vi "ConfigureQDC.vi"(5 "VME module Base Address":u32, 6 "IRQ Lvl":u16, 7 "handle":i32, 8 "error in (no error)":errorcluster, 9 "# of events before transfer (max 32)":u16, 10 "CBLT Addr":u16, 11 "Geo Addr":u16) -> (0 "error out":errorcluster, 3 "handle out":i32)   [LabVIEW 2014]
uses:
  Program Files (x86)/CAEN/Comm/labview/CAENComm.lvlib
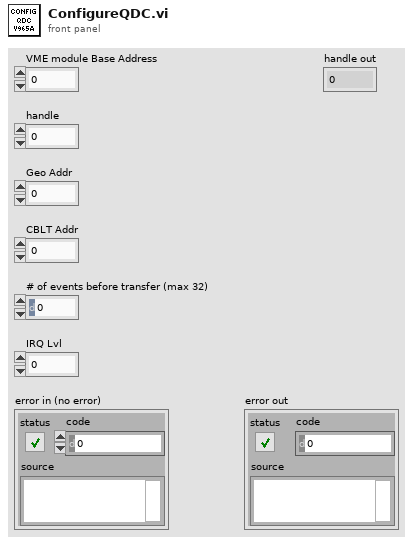
[diagram p1: front panel]
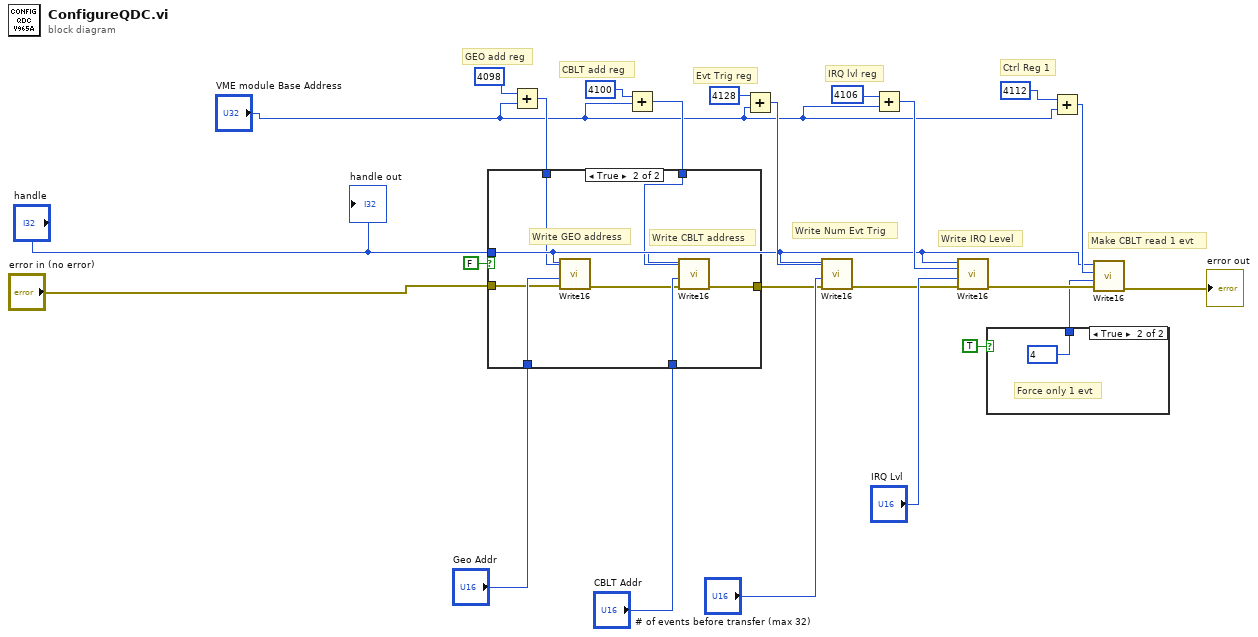
[diagram p0: block diagram]
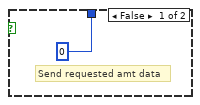
[diagram p2: hidden frame]
diagram:
  # "Ctrl Reg 1"
  # "Make CBLT read 1 evt"
  # "Evt Trig reg"
  # "Write Num Evt Trig"
  # "IRQ lvl reg"
  # "Write IRQ Level"
  # "CBLT add reg"
  # "GEO add reg"
  n1 = Add(x=u32 4098, y="VME module Base Address") -> (x+y=w11:u32)
  n2 = Add(x=u32 4100, y="VME module Base Address") -> (x+y=w15:u32)
  n3 = case shown="True" FALSE {
    tunnel: [w25 w33] -> w17
    tunnel: "CBLT Addr" -> [_ w32]
    tunnel: w15 -> [_ w31]
    tunnel: "Geo Addr" -> [_ w29]
    tunnel: w11 -> [_ w28]
    tunnel: "error in (no error)" -> [w25 w27]
    tunnel: "handle" -> [_ w26]
    frame False {
    }
    frame True {
      # "Write CBLT address"
      # "Write GEO address"
      n4 = call "Write16.vi"("error in (no error)"=w27, "Data"=w29, "Address"=w28, "handle"=w26) -> ("error out"=w30:errorcluster)  [unwired: 7 in]
      n5 = call "Write16.vi"("error in (no error)"=w30, "Data"=w32, "Address"=w31, "handle"=w26) -> ("error out"=w33:errorcluster)  [unwired: 7 in]
    }
  }
  n6 = Add(x=u32 4128, y="VME module Base Address") -> (x+y=w19:u32)
  n7 = call "Write16.vi"("error in (no error)"=w17, "Data"="# of events before transfer (max 32)", "Address"=w19, "handle"="handle") -> ("error out"=w20:errorcluster)  [unwired: 7 in]
  n8 = Add(x=u32 4106, y="VME module Base Address") -> (x+y=w22:u32)
  n9 = call "Write16.vi"("error in (no error)"=w20, "Data"="IRQ Lvl", "Address"=w22, "handle"="handle") -> ("error out"=w8:errorcluster)  [unwired: 7 in]
  n10 = case shown="True" TRUE {
    tunnel: [0 u16 4 ("Data")] -> w3
    frame False {
      # "Send requested amt data"
    }
    frame True {
      # "Force only 1 evt"
    }
  }
  n11 = Add(x=u32 4112, y="VME module Base Address") -> (x+y=w6:u32)
  n12 = call "Write16.vi"("error in (no error)"=w8, "Data"=w3, "Address"=w6, "handle"="handle") -> ("error out"=→"error out":errorcluster)  [unwired: 7 in]
  "handle out" <- "handle"
